vi "Fetch Oscilloscope trace.vi"() -> ()   [LabVIEW 2020]
uses:
  <instrlib>/Tektronix TDS 200 1000 2000 Series/Public/Data/Read (Multiple Waveforms).vi
  <vilib>/Waveform/WDTFileIO.llb/Export Waveforms To Spreadsheet File (1D).vi
  <instrlib>/Tektronix TDS 200 1000 2000 Series/Tektronix TDS 200 1000 2000 Series.lvlib
panel:
  in  "Tab Control":enum32{"Page 1", "Page 2"}(tab)
  in  "VISA resource name":refnum<visa-resource-name>
  in  "OK Button":bool
  in  "Suff channel":i32=1
  in  "Add rise/fall suffix":bool
  out "Waveform Graph":waveform(dbl)[](graph)
  in  "OK Button 2":bool
  in  "Stop Button":bool
  in  "append to file?":bool
  in  "file path (dialog if empty)":path
  out "error out":errorcluster
  in  "Channels and optional channel names":cluster{"Blank Button":bool, "String":string}[](array[cluster])=[{"Blank Button"=TRUE, "String"=""}, {"Blank Button"=FALSE, "String"=""}, {"Blank Button"=FALSE, "String"=""}, {"Blank Button"=FALSE, "String"=""}]
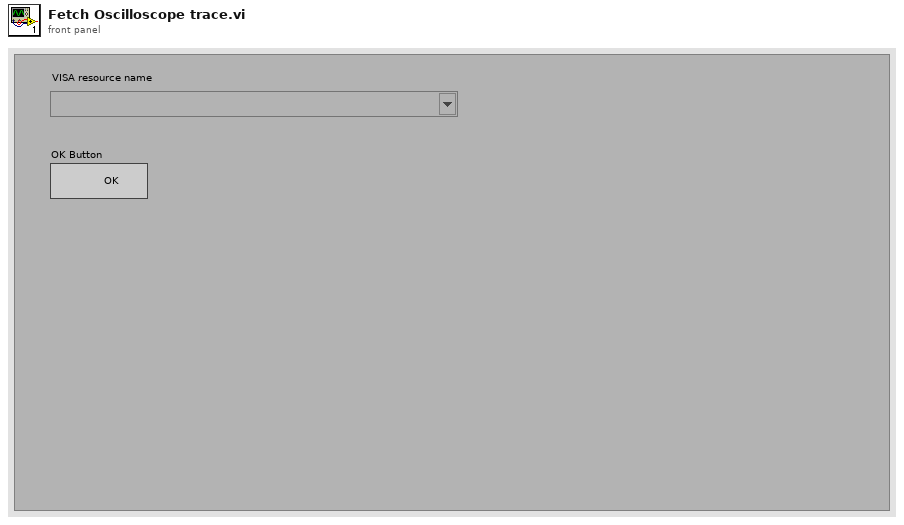
[diagram p1: front panel]
types:
  T1 = enum8{"Enabled", "Disabled", "Disabled and Grayed Out"}
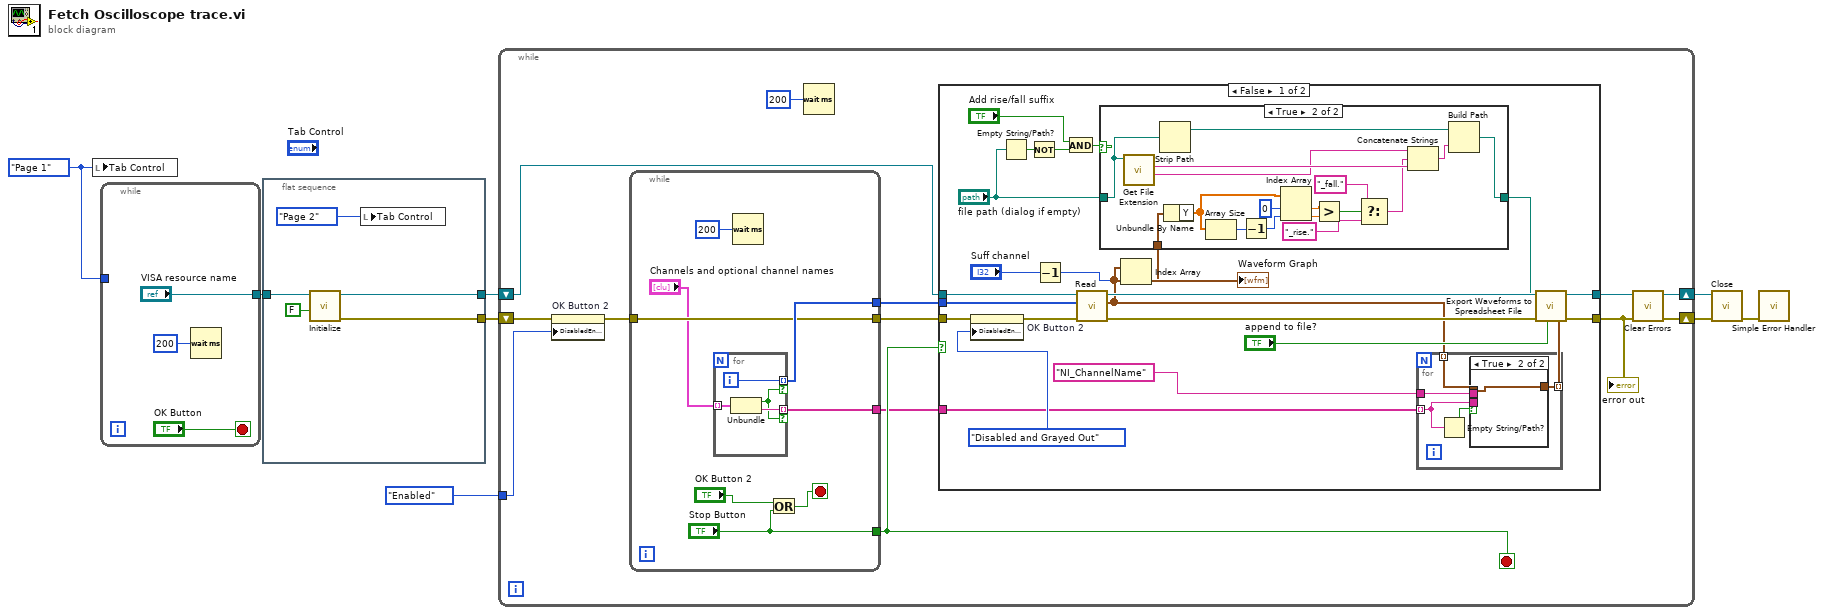
[diagram p0: block diagram]
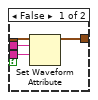
[diagram p3: hidden frame]
diagram:
  w4 = enum32{"Page 1", "Page 2"}."Page 1" ("Tab Control")
  n1 = local write "Tab Control"(w4) -> ()
  n2 = while {
    tunnel: ["VISA resource name"] -> w5
    tunnel: w4 -> [_]
    stop <- "OK Button" stop-if-true
    n3 = Wait (ms)(milliseconds to wait=u32 200) -> ()  [unwired: 1 out]
  }
  n4 = flat-sequence {
    tunnel: [w16] -> w8
    tunnel: [w15] -> w3
    tunnel: w5 -> [w14]
    frame #0 {
      n5 = call <instrlib>:"Initialize.vi"("Reset? (T: Yes)"=FALSE, "VISA resource name"=w14) -> ("error out"=w15:errorcluster, "VISA resource name out"=w16:refnum<visa-resource-name>)  [unwired: 8 in]
      n6 = local write "Tab Control"(enum32{"Page 1", "Page 2"}."Page 2" ("Tab Control")) -> ()
    }
  }
  n7 = while {
    shift-right: [w27] -> w7
    shift-left: w8 -> [w28]
    shift-right: [w21] -> w6
    shift-left: w3 -> [w20]
    tunnel: T1."Enabled" ("Disabled") -> [w18]
    stop <- w23 stop-if-true
    n8 = property on="OK Button 2" class="Bool"(error in=w20, "DisabledEnum"=w18) -> (error out=w19:errorcluster)  [unwired: 1 in, 1 out]
    n9 = while {
      tunnel: [w88] -> w26
      tunnel: [w87] -> w25
      tunnel: w19 -> [w87]
      tunnel: ["Stop Button"] -> w23
      tunnel: [w81] -> w17
      stop <- w83 stop-if-true
      n10 = for {
        tunnel: "Channels and optional channel names" -> [w91] mode=indexing
        tunnel: [w92] -> w88 mode=indexing if=w89
        tunnel: [w90] -> w81 mode=indexing if=w89
        i -> [w92]
        n11 = Unbundle(w91) -> ("Blank Button"=w89:bool, "String"=w90:string)
      }
      n12 = Wait (ms)(milliseconds to wait=u32 200) -> ()  [unwired: 1 out]
      n13 = Or(x="OK Button 2", y="Stop Button") -> (x .or. y?=w83:bool)
    }
    n14 = Wait (ms)(milliseconds to wait=u32 200) -> ()  [unwired: 1 out]
    n15 = case shown="False" w23 {
      tunnel: w28 -> [w50 w79]
      tunnel: [w49 w79] -> w27
      tunnel: w26 -> [w48 _]
      tunnel: w25 -> [w44 w80]
      tunnel: [w46 w80] -> w22
      tunnel: w17 -> [w41 _]
      frame False {
        n16 = property on="OK Button 2" class="Bool"(error in=w44, "DisabledEnum"=T1."Disabled and Grayed Out" ("Disabled")) -> (error out=w43:errorcluster)  [unwired: 1 in, 1 out]
        n17 = Empty String/Path?(string/path="file path (dialog if empty)") -> (empty?=w36:bool)
        n18 = Not(x=w36) -> (.not. x?=w35:bool)
        n19 = Decrement(x="Suff channel") -> (x-1=w30:i32)
        n20 = And(x="Add rise/fall suffix", y=w35) -> (x .and. y?=w38:bool)
        n21 = call-poly <instrlib>:"Read.vi"("error in (no error)"=w43, "Channels"=w48, "VISA resource name"=w50) -> ("error out"=w47:errorcluster, "Waveform Data"=w32:waveform(dbl)[], "VISA resource name out"=w49:refnum<visa-resource-name>)  [unwired: 6 in]
        "Waveform Graph" <- w32
        n22 = Index Array(array=w32, index=w30) -> (element=w29:waveform(dbl))
        n23 = case shown="True" w38 {
          tunnel: [w51 w60] -> w33
          tunnel: "file path (dialog if empty)" -> [w51 w58]
          tunnel: w29 -> [_ w68]
          frame False {
          }
          frame True {
            n24 = call <vilib>:"Get File Extension.vi"("file"=w58) -> ("filename without extension"=w56:string, "lowercase file extension"=w57:string)  [unwired: 6 in, 3 out]
            n25 = Strip Path(path=w58) -> (stripped path=w59:path)  [unwired: 1 out]
            n26 = Unbundle By Name(w68) -> ("Y"=w64:dbl[])
            n27 = Array Size(array=w64) -> (size(s)=w67:i32)
            n28 = Decrement(x=w67) -> (x-1=w66:i32)
            n29 = Index Array(array=w64, index #1=0 ("index"), index #2=w66) -> (element #1=w63:dbl, element #2=w62:dbl)
            n30 = Greater?(x=w63, y=w62) -> (0:w61:bool)
            n31 = Select(t="_fall.", s=w61, f="_rise.") -> (s? t:f=w54:string)
            n32 = Concatenate Strings(w56, w54, w57) -> (w55:string)
            n33 = Build Path(base path=w59, name or relative path=w55) -> (appended path=w60:path)
          }
        }
        n34 = for {
          tunnel: w32 -> [w73] mode=indexing
          tunnel: w41 -> [w70] mode=indexing
          tunnel: "NI_ChannelName" ("name") -> [w72]
          tunnel: [w71] -> w39 mode=indexing
          n35 = Empty String/Path?(string/path=w70) -> (empty?=w69:bool)
          n36 = case shown="True" w69 {
            tunnel: w73 -> [w77 w78]
            tunnel: w72 -> [w76 _]
            tunnel: [w75 w78] -> w71
            tunnel: w70 -> [w74 _]
            frame False {
              n37 = Set Waveform Attribute(5:w74, 6:w76, 7:w77) -> (3:w75:waveform(dbl))  [unwired: 1 in, 2 out]
            }
            frame True {
            }
          }
        }
        n38 = call-poly <vilib>:"Export Waveforms to Spreadsheet File.vi"("append to file? (new file:F)"="append to file?", "error in (no error)"=w47, "waveforms"=w39, "file path (dialog if empty)"=w33) -> ("error out"=w46:errorcluster)  [unwired: 6 in, 1 out]
      }
      frame True {
      }
    }
    "error out" <- w22
    n39 = call <vilib>:"Clear Errors.vi"("error in (no error)"=w22) -> ("error out"=w21:errorcluster)  [unwired: 5 in, 1 out]
  }
  n40 = call <instrlib>:"Close.vi"("error in (no error)"=w6, "VISA resource name"=w7) -> ("error out"=w2:errorcluster)  [unwired: 9 in]
  n41 = call <vilib>:"Simple Error Handler.vi"("error in (no error)"=w2) -> ()  [unwired: 4 in, 5 out]
